vi "AreaCheck.vi"(0 "Vision_Image In":T3(plugin-control), 5 "List ROI Ref":refnum<vi>, 7 "AlgIn":T4, 11 "error in (no error)":errorcluster, 12 "ParameterIn":string, 14 "RootPath":path) -> (6 "ParameerOut":string, 10 "Cancel?":bool, 15 "error out":errorcluster)   [LabVIEW 2019]
uses:
  Controls/V_Analysis_Type.ctl
  Controls/_UI Command Cluster/Pattern Match_UI Command.ctl
  <vilib>/Utility/miscctls.llb/LVPointTypeDef.ctl
  Controls/Area Check/Area Check_Parameter.ctl
  Controls/Analysis_Setting.ctl
  <vilib>/vision/Image Controls.llb/IMAQ Image.ctl
  11e1650d-9a27-4c98-b785-94bb4e51b252.vi
  fe4c8c9f-3b30-4d10-b5c7-71603a67618a.vi
  7765c890-54c4-40a3-a063-9b2138e01ba1.vi
  ff688e6c-f413-41b3-9d93-3794729c7324.vi
  <vilib>/JDP Science/JSONtext/JSON text to Variant.vi
  <vilib>/JDP Science/JSONtext/Variant to JSON Text.vi
  <vilib>/userdefined/High Color/IMAQdx.ctl
  <vilib>/vision/NI_Vision_Development_Module.lvlib
panel:
  out "AreaDataOut":T2(array[cluster]) {"AreaDataOut"."Rectangle"."Rotation" format="%.2f"; "AreaDataOut"."Rectangle"."Left" scale=0.0..1024.0; "AreaDataOut"."Rectangle"."Right" scale=0.0..1024.0}
  in  "Run Algorithm":bool
  out "Image":T3(plugin-control)
  out "Algout":T4=enum."G_PatternMatching"
  in  "SetROI":bool
  in  "Cancel":bool
  in  "Done":bool
  in  "PatternMatchTab":T5(tab)
  in  "NoItem":dbl=1.0 caption="無料(少料)百分比" min=1.0 max=100.0 step=1.0
  out "Check Type":T6(ring) caption="判斷型態"
  in  "Table Control":string[][](table)
  # "%"
  # "以下(Under)"
  # "全畫面(Total Area)"
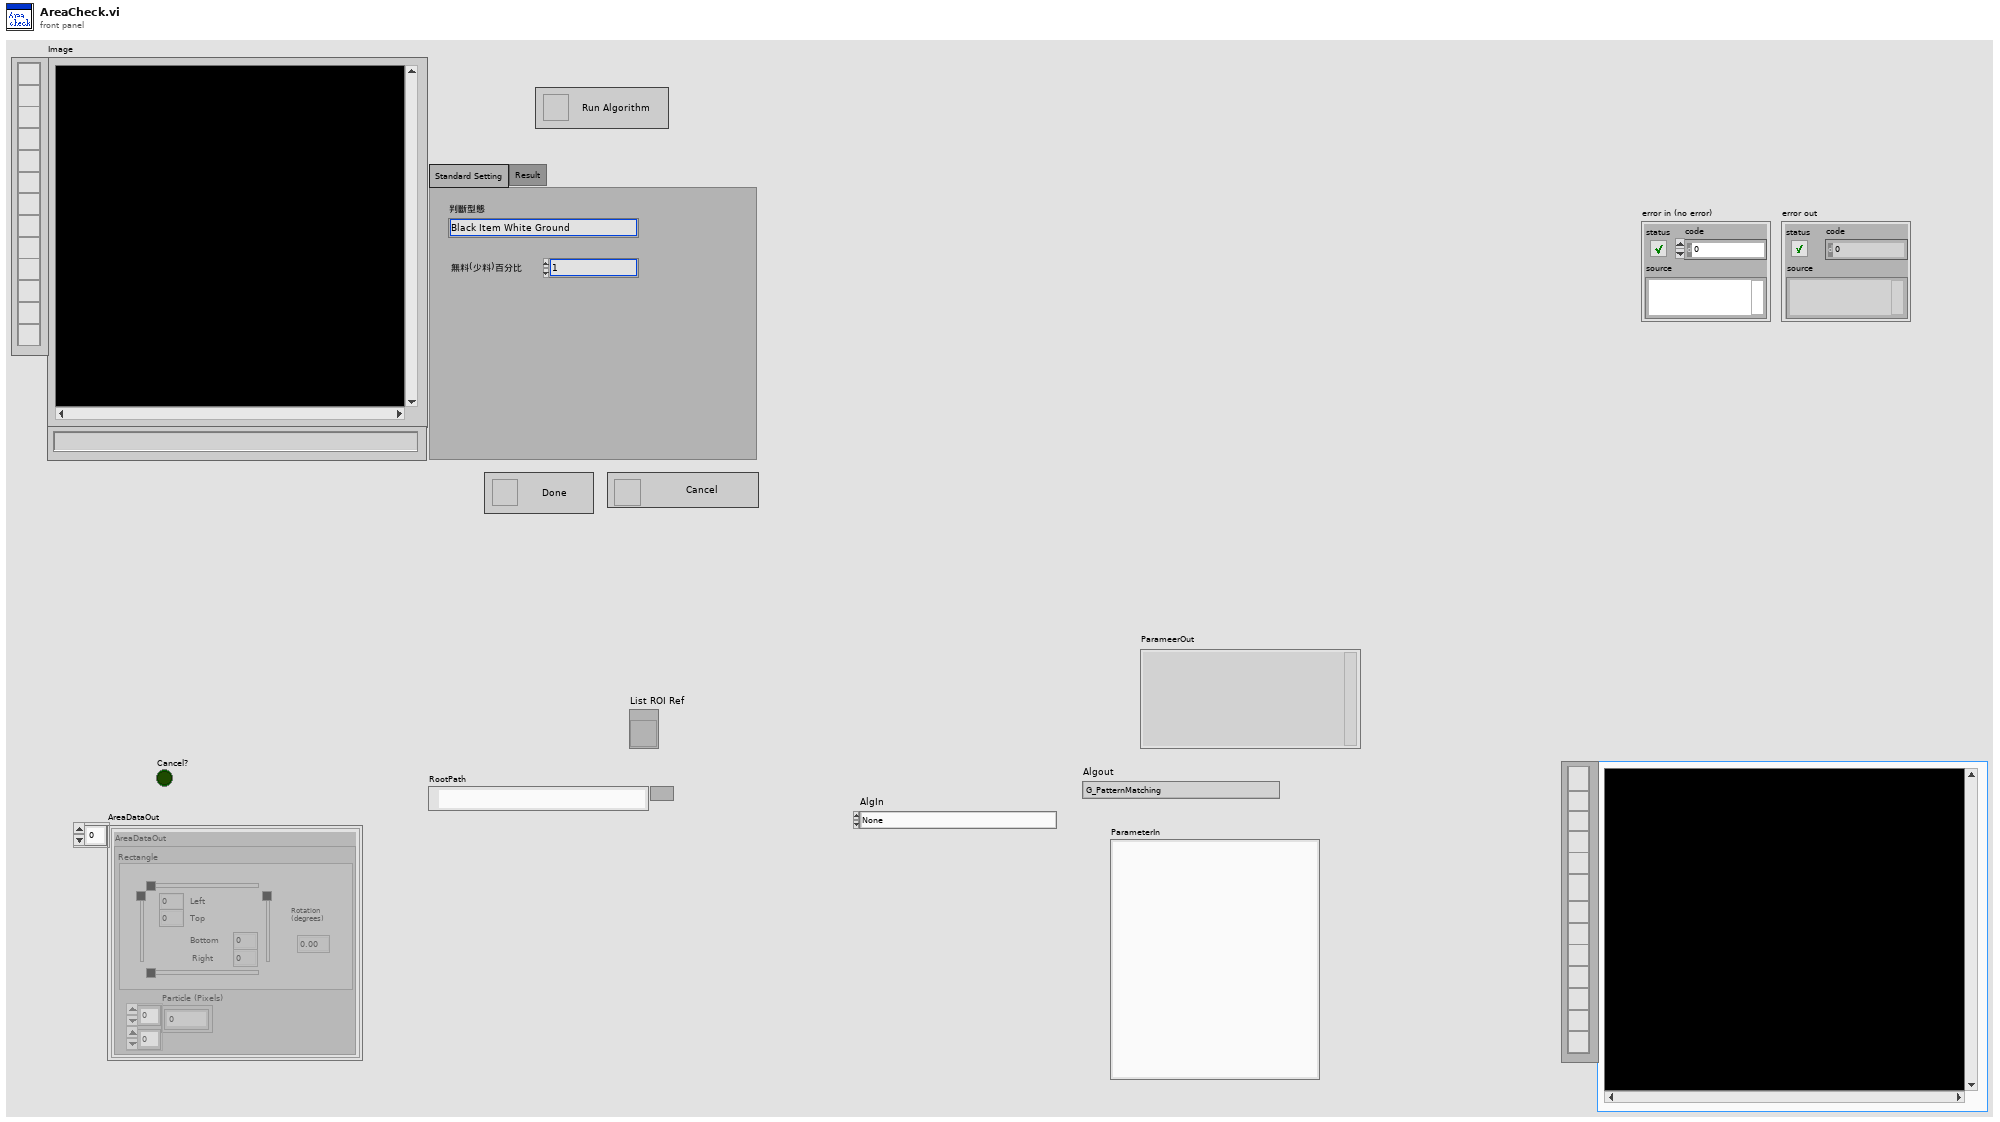
[diagram p1: front panel]
types:
  T1 = typedef "IMAQ Rectangle" = cluster{"Left":i32, "Top":i32, "Right":i32, "Bottom":i32, "Rotation":dbl}
  T2 = cluster{"AreaDataOut":cluster{"Rectangle":T1, "Particle (Pixels)":dbl[][]}}[]
  T3 = typedef "IMAQ Image.ctl" = refnum<image>
  T4 = typedef "V_Analysis_Type.ctl" = enum16{"None", "C_Color Pattern Matching", "G_PatternMatching", "G_ShapeDectect", "G_GeometricMatch", "B_Area Check"}
  T5 = enum32{"Standard Setting", "Advanced Setting", "Result"}
  T6 = enum16{"Black Item White Ground", "White Item Black Ground"}
  T7 = typedef "Image Type" = u32
  T8 = typedef "Pattern Match_UI Command.ctl" = enum16{"Init", "Done", "Cancel", "RunAlgorithm", "SetTemplate", "SetROI", "ClearOverlay", "Load Template", "Draw Overlay", "Offset", "Draw Curve"}
  T9 = typedef "LVPointTypeDef.ctl" = cluster{"Horizontal":i16, "Vertical":i16}
  T10 = typedef "IMAQdx.ctl" = refnum<k21>
  T11 = typedef "Area Check_Parameter.ctl" = cluster{"Check Type":enum16{"Black Item White Ground", "White Item Black Ground"}, "NoItem":dbl}
  T12 = cluster{"Global Rectangle":i32[], "Contours":cluster{"Contour Type":u32, "ROI Type":u32, "Points":i32[]}[]}
  T13 = typedef "Analysis_Setting.ctl" = cluster{"PreProcess":T4, "Parameter":string}
  T14 = cluster{"AreaDataOut":cluster{"Rectangle":T1, "Particle Measurements (Pixels)":dbl[][]}}[]
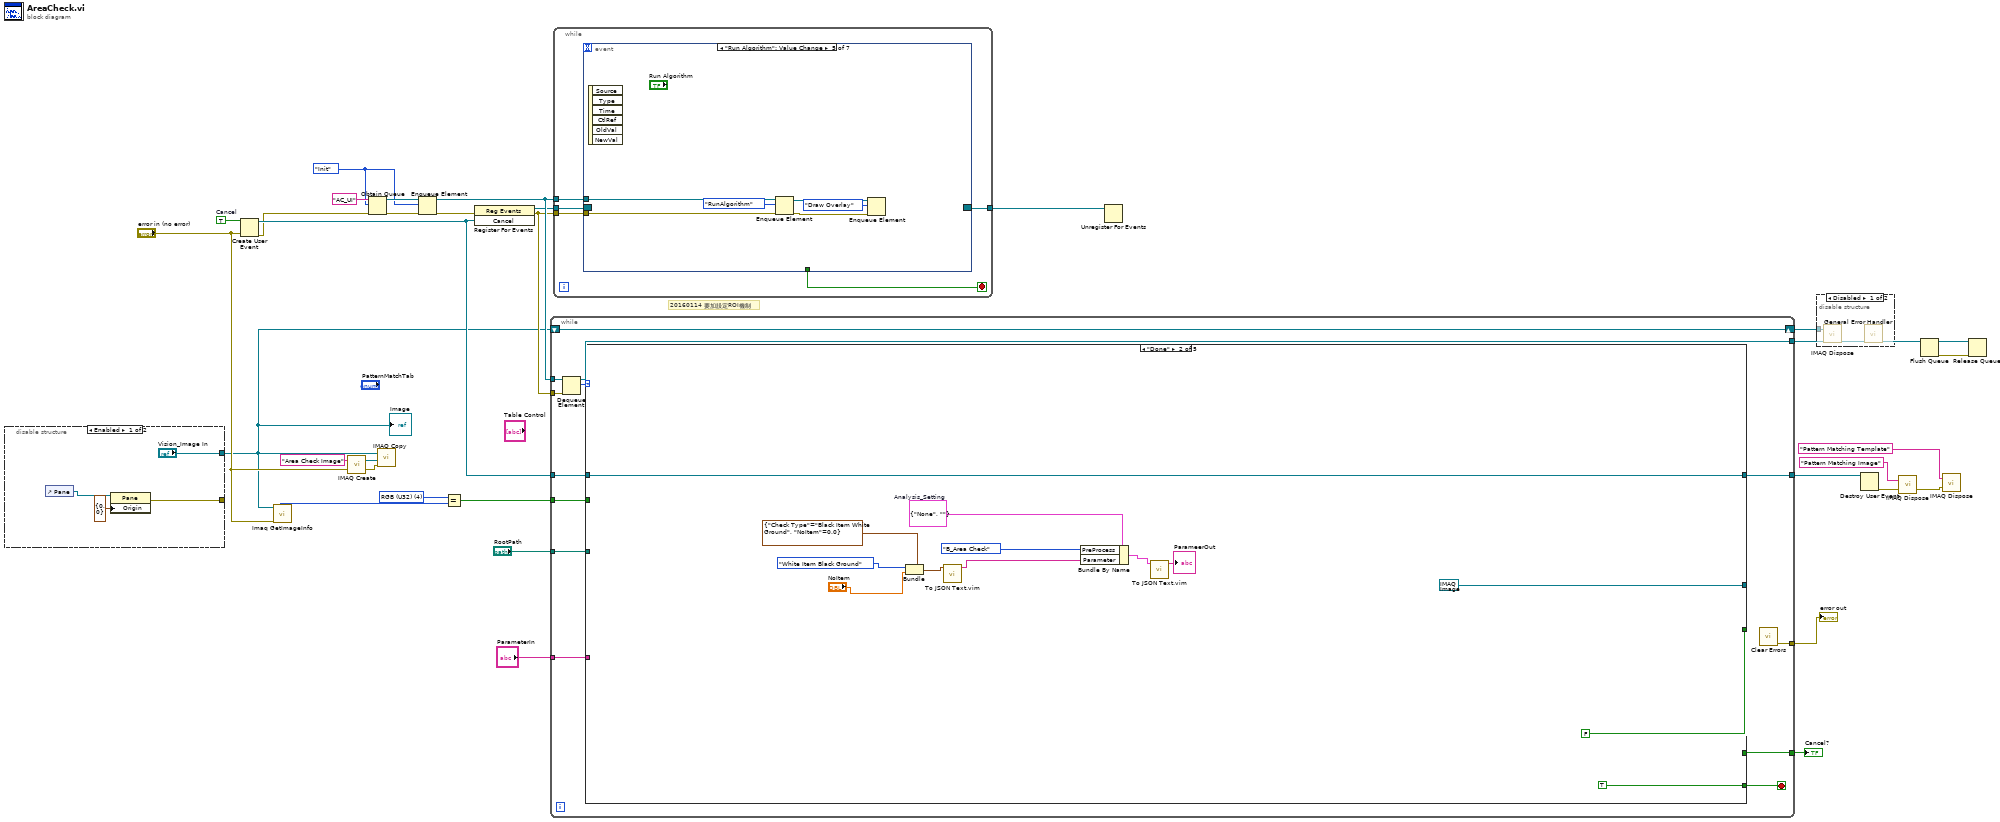
[diagram p0: block diagram]
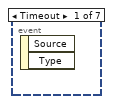
[diagram p2: hidden frame]
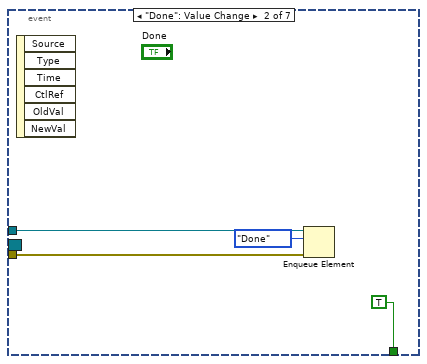
[diagram p3: hidden frame]
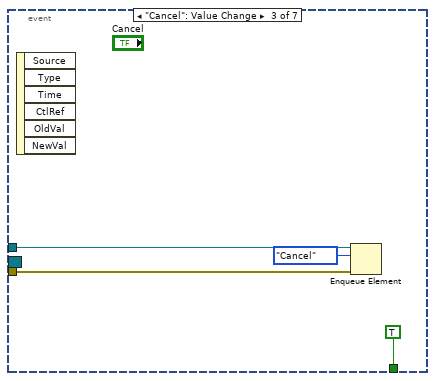
[diagram p4: hidden frame]
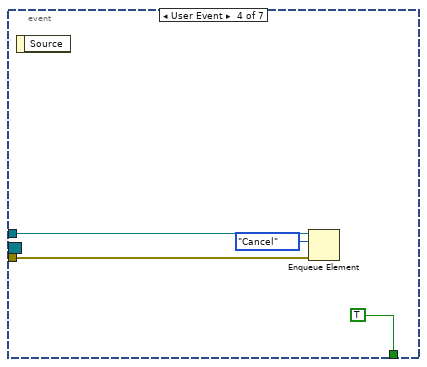
[diagram p5: hidden frame]
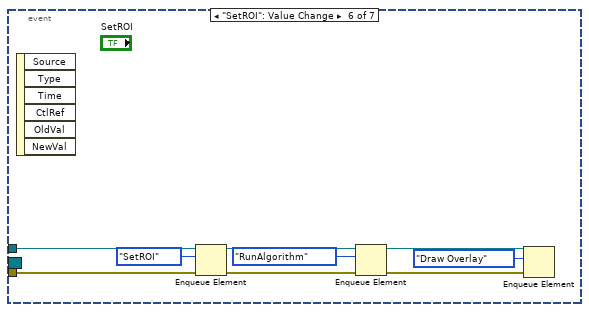
[diagram p6: hidden frame]
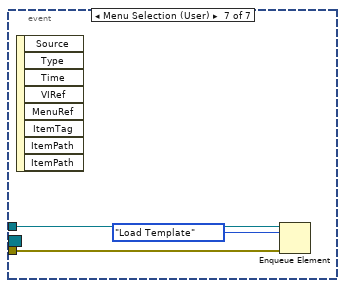
[diagram p7: hidden frame]
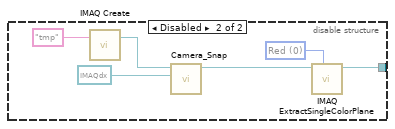
[diagram p8: hidden frame]
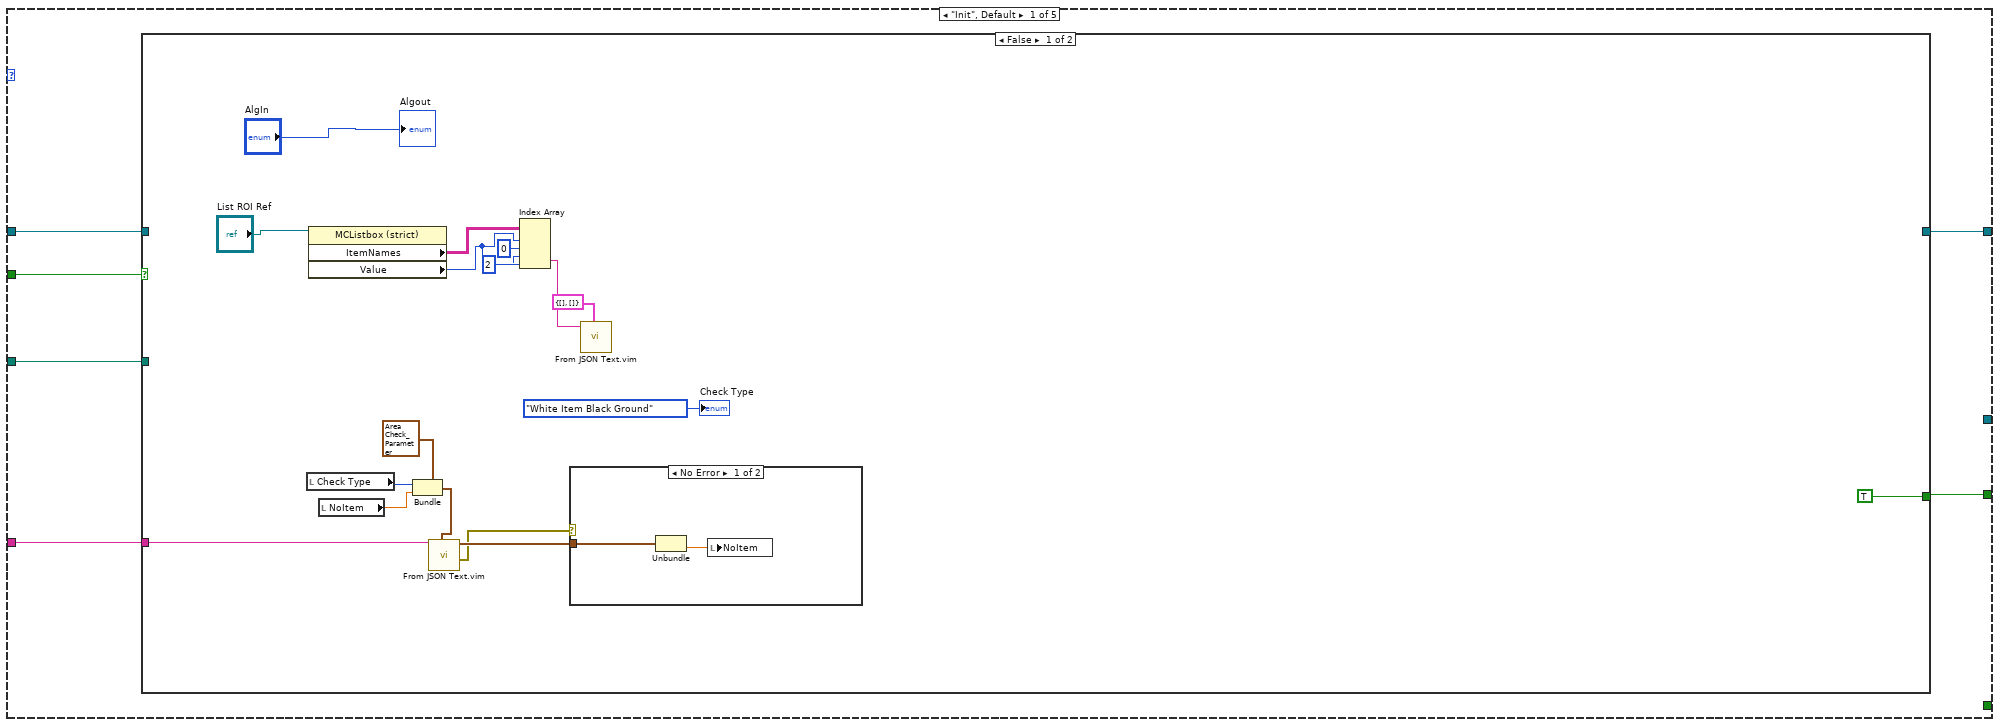
[diagram p10: hidden frame]
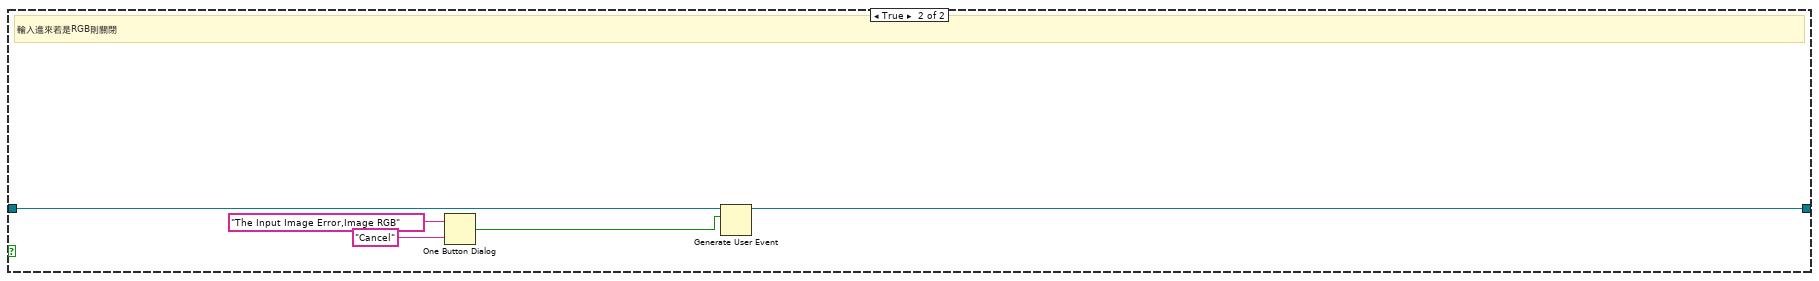
[diagram p12: hidden frame]
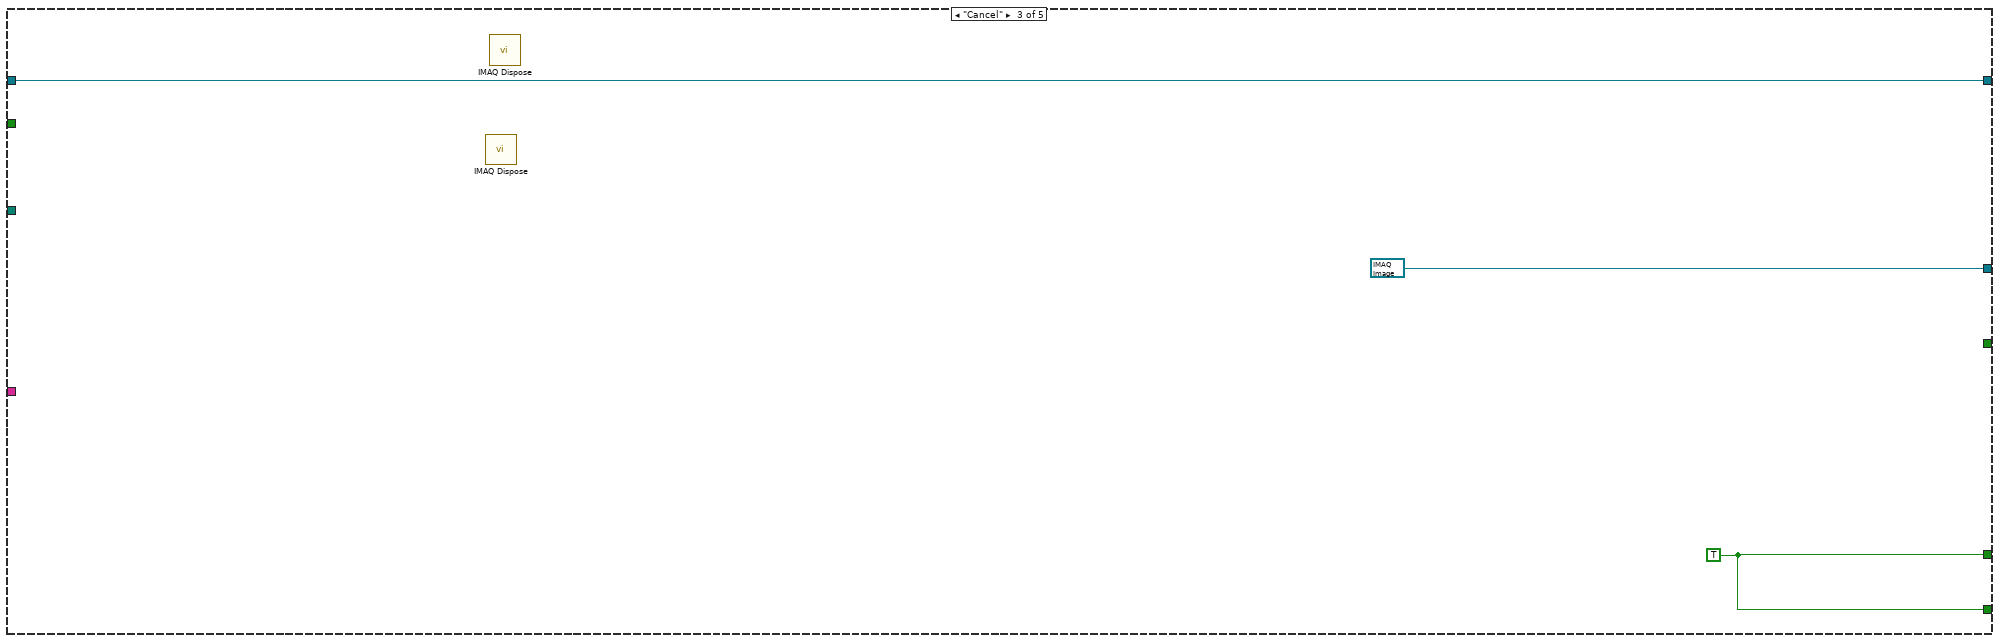
[diagram p13: hidden frame]
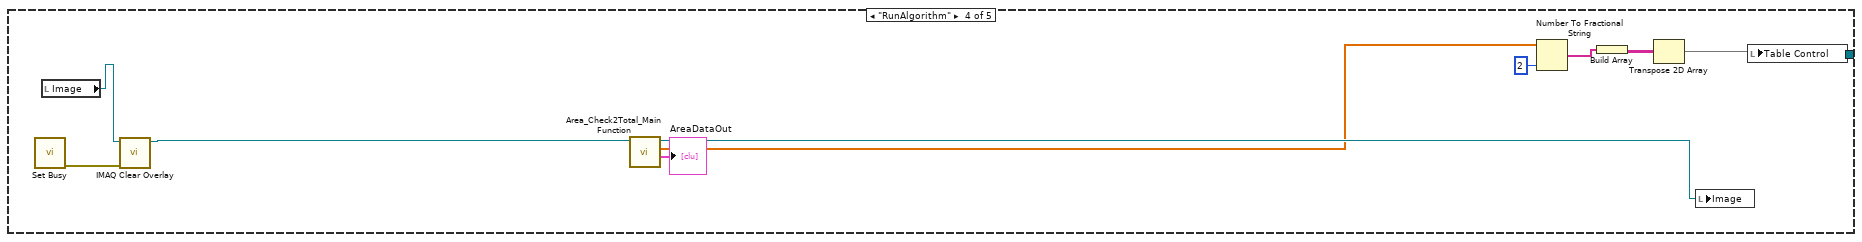
[diagram p14: hidden frame]
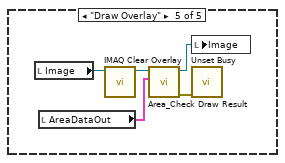
[diagram p15: hidden frame]
diagram:
  w18 = TRUE  # Cancel
  w20 = T7 4 items=["Grayscale (U8)", "Grayscale (I16)", "Grayscale (SGL)", "Complex (CSG)", "RGB (U32)", "HSL (U32)", "RGB (U64)", "Grayscale (U16)"] ("x")
  w19 = Pattern_Match_UI_Command."Init"
  # "20160114 要加設定ROI機制"
  n1 = disable-structure shown="Enabled" {
    disable-tunnel: ["Vision_Image In" w39] -> w1
    disable-tunnel: [w34 _] -> _
    frame Enabled {
      n2 = control-ref of="Pane"() -> (w36:refnum<vi>)
      n3 = property class="Pane"(reference=w36, "Origin"=T9 {"Horizontal"=0, "Vertical"=0}) -> (error out=w34:errorcluster)  [unwired: 1 in, 1 out]
    }
    frame Disabled {
      w38 = 0 items=["Red", "Green", "Blue", "Hue", "Saturation", "Luminance", "Value", "Intensity"] ("Color Plane")
      n4 = call "IMAQ Create"("Image Name"="tmp") -> ("New Image"=w41:T3)  [unwired: 4 in, 1 out]
      n5 = call "Camera_Snap.vi"("Camera Session In"=T10 refnum, "Image In"=w41) -> ("New Image"=w40:T3)  [unwired: 8 in, 1 out]
      n6 = call "IMAQ ExtractSingleColorPlane"("Color Plane"=w38, "Image Src"=w40) -> ("Image Dst Out"=w39:T3)  [unwired: 2 in, 7 out]
    }
  }
  "Image" <- w1
  n7 = Create User Event(user event datatype=w18, error in="error in (no error)") -> (user event=w15:refnum<user-event>, error out=w6:errorcluster)
  n8 = call "Imaq GetImageInfo"("error in (no error)"="error in (no error)", "Image"=w1) -> ("Image Type"=w21:T7)  [unwired: 2 in, 7 out]
  n9 = call "IMAQ Create"("Image Name"="Area Check Image", "error in (no error)"="error in (no error)") -> ("New Image"=w30:T3, "error out"=w5:errorcluster)  [unwired: 3 in]
  n10 = Obtain Queue(name (unnamed)="AC_UI", element data type=w19, error in (no error)=w6) -> (queue out=w28:refnum<queue>, error out=w27:errorcluster)  [unwired: 2 in, 1 out]
  n11 = call "IMAQ Copy"("error in (no error)"=w5, "Image Dst"=w30, "Image Src"=w1) -> ()  [unwired: 3 in, 2 out]
  n12 = Enqueue Element(queue=w28, element=w19, error in (no error)=w27) -> (queue out=w24:refnum<queue>, error out=w12:errorcluster)  [unwired: 1 in, 1 out]
  n13 = Equal?(x=w20, y=w21) -> (x = y?=w16:bool)
  n14 = register-events(error in=w12, w15) -> (reference out=w17:refnum<event-registration>, error out=w11:errorcluster)  [unwired: 1 in]
  n15 = while {
    shift-right: [w56] -> w33
    shift-left: w1 -> [w56]
    tunnel: [w55] -> w32
    tunnel: w24 -> [w53]
    tunnel: w11 -> [w51]
    tunnel: [w50] -> w23
    tunnel: "RootPath" -> [w49]
    tunnel: w16 -> [w48]
    tunnel: w15 -> [w47]
    tunnel: [w46] -> w14
    tunnel: [w45] -> w3
    tunnel: "ParameterIn" -> [w44]
    stop <- w54 stop-if-true
    n16 = Dequeue Element(queue=w53, error in (no error)=w51) -> (queue out=w50:refnum<queue>, element=w52:T8)  [unwired: 1 in, 2 out]
    n17 = case shown="\"Done\"" w52 {
      tunnel: [_ TRUE w102 _ _] -> w54
      tunnel: [_ _ w102 _ _] -> w55
      tunnel: [_ T3 refnum ("Template Out") T3 refnum ("Template Out") _ _] -> _
      tunnel: [w62 FALSE _ _ _] -> _
      tunnel: w49 -> [w61 _ _ _ _]
      tunnel: w48 -> [w60 _ _ _ _]
      tunnel: w47 -> [w59 w94 w100 _ _]
      tunnel: [w58 w94 w100 _ _] -> w46
      tunnel: w44 -> [w57 _ _ _ _]
      frame "Init", Default {
        n18 = case shown="False" w60 {
          tunnel: [TRUE _] -> w62
          tunnel: w61 -> [_ _]
          tunnel: w59 -> [_ w84]
          tunnel: [_ w82] -> w58
          tunnel: w57 -> [w70 _]
          frame False {
            n19 = local read "Check Type"() -> (w67:T6)
            n20 = property class="MCListbox (strict)"(reference="List ROI Ref") -> ("ItemNames"=w74:string[][], "Value"=w73:i32)  [unwired: 1 in, 2 out]
            n21 = local read "NoItem"() -> (w68:dbl)
            n22 = Bundle(cluster=T11 {"Check Type"=enum."Black Item White Ground", "NoItem"=0.0}, "Check Type"=w67, "NoItem"=w68) -> (w66:T11)
            n23 = call "From JSON Text.vim"("Data Type and Default Value"=w66, "JSON"=w70) -> ("error out"=w64:errorcluster, "Data out"=w65:T11)  [unwired: 8 in]
            n24 = Index Array(array=w74, index (row) #1=w73, index (col) #1=0 ("disabled index (col)"), index (row) #2=w73, index (col) #2=2 ("disabled index (col)")) -> (element #2=w71:string)  [unwired: 1 out]
            n25 = case shown="No Error" w64 {
              tunnel: w65 -> [w81 _]
              frame No Error {
                n26 = Unbundle(w81) -> ("NoItem"=w80:dbl)  [unwired: 1 out]
                n27 = local write "NoItem"(w80) -> ()
              }
              frame Error {
              }
            }
            n28 = call "From JSON Text.vim"("Data Type and Default Value"=T12 {"Global Rectangle"=[], "Contours"=[]} ("ROI"), "JSON"=w71) -> ()  [unwired: 8 in, 2 out]
            "Algout" <- "AlgIn"
            "Check Type" <- T6."White Item Black Ground" ("Check Type")
          }
          frame True {
            # "輸入進來若是RGB則關閉"
            n29 = One Button Dialog(message="The Input Image Error,Image RGB", button name ("OK")="Cancel") -> (true=w83:bool)
            n30 = Generate User Event(user event=w84, event data cluster=w83) -> (user event out=w82:refnum<user-event>)  [unwired: 2 in, 1 out]
          }
        }
      }
      frame "Done" {
        w97 = T13 {"PreProcess"=enum."None", "Parameter"=""}  # Analysis_Setting
        n31 = Bundle(cluster=T11 {"Check Type"=enum."Black Item White Ground", "NoItem"=0.0}, "Check Type"=T6."White Item Black Ground", "NoItem"="NoItem") -> (w89:T11)
        n32 = call "To JSON Text.vim"("Anything"=w89) -> ("<JSON>"=w93:string)  [unwired: 9 in, 1 out]
        n33 = Bundle By Name(cluster=w97, "PreProcess"=V_Analysis_Type."B_Area Check" ("Analysis"), "Parameter"=w93) -> (w92:T13)
        n34 = call "To JSON Text.vim"("Anything"=w92) -> ("<JSON>"=→"ParameerOut":string)  [unwired: 9 in, 1 out]
      }
      frame "Cancel" {
        w102 = TRUE
        n35 = call "IMAQ Dispose"() -> ()  [unwired: 6 in, 1 out]
        n36 = call "IMAQ Dispose"() -> ()  [unwired: 6 in, 1 out]
      }
      frame "RunAlgorithm" {
        n37 = call <vilib>:"Set Busy.vi"() -> ("error out"=w112:errorcluster)  [unwired: 10 in, 1 out]
        n38 = local read "Image"() -> (w111:T3)
        n39 = call "IMAQ Clear Overlay"("error in (no error)"=w112, "Image"=w111) -> ("Image Out"=w104:T3)  [unwired: 8 in, 1 out]
        n40 = call "Area_Check2Total_Main Function.vi"("img in"=w104) -> ("AreaDataOut"=→"AreaDataOut":T14, "Array"=w105:dbl[], "Iimg out"=w109:T3)  [unwired: 7 in, 1 out]
        n41 = Number To Fractional String(number=w105, precision (6)=i16 2) -> (F-format string=w108:string[])  [unwired: 2 in]
        n42 = Build Array(w108) -> (w107:string[][])
        n43 = Transpose 2D Array(2D array=w107) -> (transposed array=w106:string[][])
        n44 = local write "Image"(w109) -> ()
        n45 = local write "Table Control"(w106) -> ()
      }
      frame "Draw Overlay" {
        n46 = local read "Image"() -> (w116:T3)
        n47 = local read "AreaDataOut"() -> (w117:T2)
        n48 = call "IMAQ Clear Overlay"("Image"=w116) -> ("Image Out"=w115:T3)  [unwired: 9 in, 1 out]
        n49 = call "Area_Check Draw Result.vi"("AreaDataOut"=w117, "Refnum in"=w115) -> ("error out"=w113:errorcluster, "Refnum out"=w114:T3)  [unwired: 8 in]
        n50 = local write "Image"(w114) -> ()
        n51 = call <vilib>:"Unset Busy.vi"("error in (no error)"=w113) -> ()  [unwired: 10 in, 1 out]
      }
    }
    n52 = call <vilib>:"Clear Errors.vi"() -> ("error out"=w45:errorcluster)  [unwired: 6 in, 1 out]
  }
  "error out" <- w3
  "Cancel?" <- w32
  n53 = while {
    tunnel: w24 -> [w121]
    tunnel: w11 -> [w120]
    tunnel: w17 -> [w119]
    tunnel: [w118] -> w13
    stop <- w122 stop-if-true
    n54 = event shown="[4] \"Run Algorithm\": Value Change" {
      selector: w119 -> [_ _ _ _ _ _ _]
      dyn-events: [_ _ _ _ _ _ _] -> w118
      timeout: _ -> [_ _ _ _ _ _ _]
      tunnel: [_ TRUE TRUE TRUE _ _ _] -> w122
      tunnel: w121 -> [_ w125 w129 w133 w140 w149 w152]
      tunnel: w120 -> [_ w124 w128 w132 w139 w148 w151]
      event Timeout {
        n55 = event-data() -> ()  [unwired: 1 in, 2 out]
      }
      event "Done": Value Change {
        n56 = event-data() -> ()  [unwired: 1 in, 6 out]
        n57 = Enqueue Element(queue=w125, element=Pattern_Match_UI_Command."Done", error in (no error)=w124) -> ()  [unwired: 1 in, 3 out]
      }
      event "Cancel": Value Change {
        n58 = event-data() -> ()  [unwired: 1 in, 6 out]
        n59 = Enqueue Element(queue=w129, element=Pattern_Match_UI_Command."Cancel", error in (no error)=w128) -> ()  [unwired: 1 in, 3 out]
      }
      event User Event {
        n60 = event-data() -> ()  [unwired: 1 in, 1 out]
        n61 = Enqueue Element(queue=w133, element=Pattern_Match_UI_Command."Cancel", error in (no error)=w132) -> ()  [unwired: 1 in, 3 out]
      }
      event "Run Algorithm": Value Change {
        n62 = event-data() -> ()  [unwired: 1 in, 6 out]
        n63 = Enqueue Element(queue=w140, element=Pattern_Match_UI_Command."RunAlgorithm", error in (no error)=w139) -> (queue out=w137:refnum<queue>, error out=w135:errorcluster)  [unwired: 1 in, 1 out]
        n64 = Enqueue Element(queue=w137, element=Pattern_Match_UI_Command."Draw Overlay", error in (no error)=w135) -> ()  [unwired: 1 in, 3 out]
      }
      event "SetROI": Value Change {
        n65 = event-data() -> ()  [unwired: 1 in, 6 out]
        n66 = Enqueue Element(queue=w149, element=Pattern_Match_UI_Command."SetROI", error in (no error)=w148) -> (queue out=w146:refnum<queue>, error out=w145:errorcluster)  [unwired: 1 in, 1 out]
        n67 = Enqueue Element(queue=w146, element=Pattern_Match_UI_Command."RunAlgorithm", error in (no error)=w145) -> (queue out=w142:refnum<queue>, error out=w143:errorcluster)  [unwired: 1 in, 1 out]
        n68 = Enqueue Element(queue=w142, element=Pattern_Match_UI_Command."Draw Overlay", error in (no error)=w143) -> ()  [unwired: 1 in, 3 out]
      }
      event Menu Selection (User) {
        n69 = event-data() -> ()  [unwired: 1 in, 8 out]
        n70 = Enqueue Element(queue=w152, element=Pattern_Match_UI_Command."Load Template", error in (no error)=w151) -> ()  [unwired: 1 in, 3 out]
      }
    }
  }
  n71 = Unregister For Events(event registration refnum=w13) -> ()  [unwired: 1 in, 1 out]
  n72 = disable-structure shown="Disabled" {
    disable-tunnel: w33 -> [w153 _]
    frame Disabled {
      n73 = call "IMAQ Dispose"("Image"=w153) -> ("error out"=w154:errorcluster)  [unwired: 5 in]
      n74 = call <vilib>:"General Error Handler.vi"("error in (no error)"=w154) -> ()  [unwired: 2 in, 13 out]
    }
    frame Enabled {
    }
  }
  n75 = Destroy User Event(user event=w14) -> (error out=w10:errorcluster)  [unwired: 1 in]
  n76 = call "IMAQ Dispose"("Image"="Pattern Matching Image" ("Image Name"), "error in (no error)"=w10) -> ("error out"=w8:errorcluster)  [unwired: 4 in]
  n77 = Flush Queue(queue=w23) -> (queue out=w26:refnum<queue>, error out=w25:errorcluster)  [unwired: 1 in, 1 out]
  n78 = call "IMAQ Dispose"("Image"="Pattern Matching Template" ("Image Name"), "error in (no error)"=w8) -> ()  [unwired: 4 in, 1 out]
  n79 = Release Queue(queue=w26, error in (no error)=w25) -> ()  [unwired: 1 in, 3 out]
